vi "CMWFetchSISOdata.vi"(8 "error in (no error)":errorcluster, 11 "VISA Refnum in":refnum<visa-resource-name>) -> (0 "error out":errorcluster, 2 "EBLer":dbl[][](array[numeric]), 3 "VISA Refnum out":refnum<visa-resource-name>)   [LabVIEW 2013]
panel:
  out "State":string
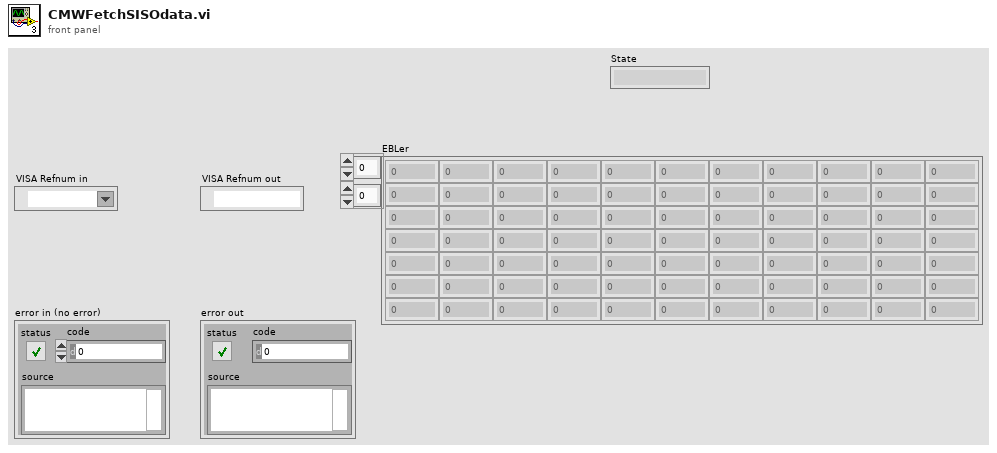
[diagram p1: front panel]
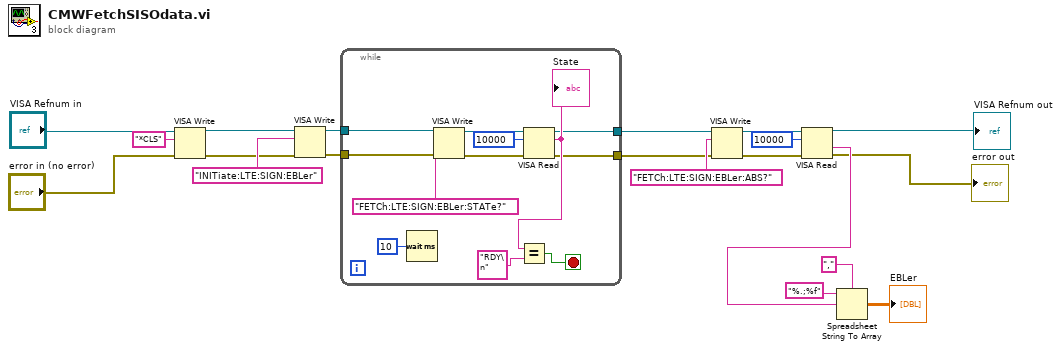
[diagram p0: block diagram]
diagram:
  n1 = VISA Write(VISA resource name="VISA Refnum in", write buffer="*CLS", error in (no error)="error in (no error)") -> (VISA resource name out=w3:refnum<visa-resource-name>, error out=w4:errorcluster)  [unwired: 1 out]
  n2 = VISA Write(VISA resource name=w3, write buffer="INITiate:LTE:SIGN:EBLer", error in (no error)=w4) -> (VISA resource name out=w9:refnum<visa-resource-name>, error out=w8:errorcluster)  [unwired: 1 out]
  n3 = while {
    tunnel: w9 -> [w25]
    tunnel: w8 -> [w24]
    tunnel: [w23] -> w7
    tunnel: [w22] -> w6
    stop <- w26 stop-if-true
    n4 = Wait (ms)(milliseconds to wait=u32 10) -> ()  [unwired: 1 out]
    n5 = VISA Write(VISA resource name=w25, write buffer="FETCh:LTE:SIGN:EBLer:STATe?", error in (no error)=w24) -> (VISA resource name out=w30:refnum<visa-resource-name>, error out=w31:errorcluster)  [unwired: 1 out]
    n6 = VISA Read(VISA resource name=w30, byte count=u32 10000, error in (no error)=w31) -> (VISA resource name out=w23:refnum<visa-resource-name>, read buffer=w28:string, error out=w22:errorcluster)  [unwired: 1 out]
    "State" <- w28
    n7 = Equal?(x=w28, y="RDY\n") -> (x = y?=w26:bool)
  }
  n8 = VISA Write(VISA resource name=w7, write buffer="FETCh:LTE:SIGN:EBLer:ABS?", error in (no error)=w6) -> (VISA resource name out=w18:refnum<visa-resource-name>, error out=w19:errorcluster)  [unwired: 1 out]
  n9 = VISA Read(VISA resource name=w18, byte count=u32 10000, error in (no error)=w19) -> (VISA resource name out=→"VISA Refnum out":refnum<visa-resource-name>, read buffer=w14:string, error out=→"error out":errorcluster)  [unwired: 1 out]
  n10 = Spreadsheet String To Array(delimiter (Tab)=",", format string="%.;%f", spreadsheet string=w14) -> (array=→"EBLer":dbl[][])  [unwired: 1 in]
